vi "removed commented lines).vi"(1 "Array in":string[](array[string])) -> (0 "Array out":string[](array[string]))   [LabVIEW 2016]
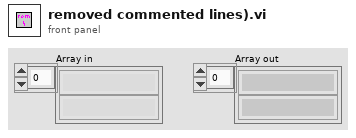
[diagram p1: front panel]
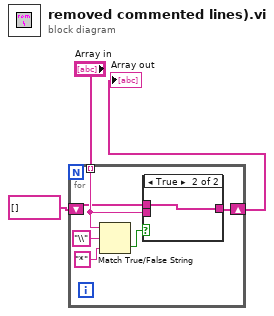
[diagram p0: block diagram]
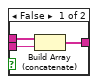
[diagram p2: hidden frame]
diagram:
  n1 = for {
    tunnel: "Array in" -> [w8] mode=indexing
    shift-right: [w7] -> w3
    shift-left: string[] [] -> [w6]
    n2 = Match True/False String(2:"*" ("false string"), 3:"\\" ("true string"), 4:w8) -> (0:w9:bool)  [unwired: 1 out]
    n3 = case shown="True" w9 {
      tunnel: w8 -> [w12 _]
      tunnel: [w10 w13] -> w7
      tunnel: w6 -> [w11 w13]
      frame False {
        n4 = Build Array (concatenate)(w11, w12) -> (w10:string[])
      }
      frame True {
      }
    }
  }
  "Array out" <- w3
